vi "Create Data Class.vi"(8 "error in (no error)":errorcluster) -> (0 "error out":errorcluster, 3 "DVR":refnum<data-value>)   [LabVIEW 2022 SP3, in "XY Stage Data Class.lvclass"]
uses:
  XY Stage Data Class.lvclass
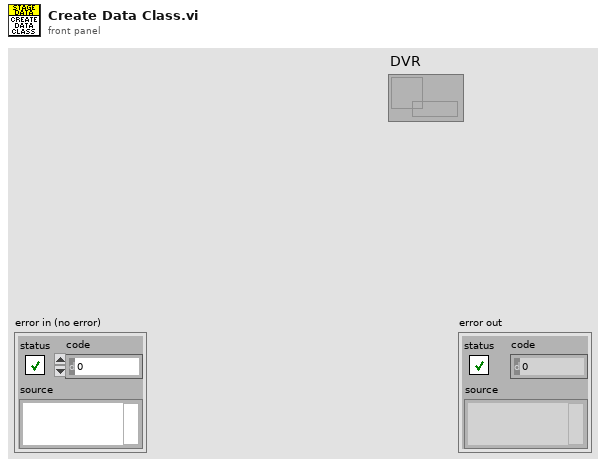
[diagram p1: front panel]
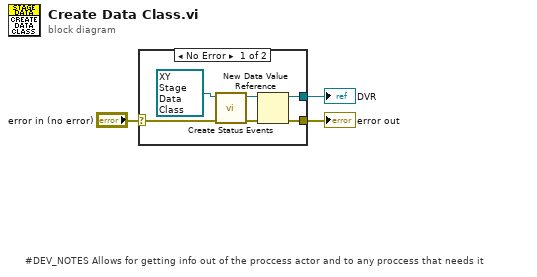
[diagram p0: block diagram]
diagram:
  # "#DEV_NOTES Allows for getting info out of the proccess actor and to any proccess that needs it"
  n1 = case shown="No Error" "error in (no error)" {
    selector: "error in (no error)" -> [w5 w10]
    tunnel: [w8 w10] -> w2
    tunnel: [w7 _] -> w1
    frame No Error {
      n2 = call "Create Status Events.vi"("error in (no error)"=w5, "XY Stage Data Class in"=refnum<class "XY Stage Data Class.lvclass"> refnum) -> ("error out"=w4:errorcluster, "XY Stage Data Class out"=w6:refnum<class "XY Stage Data Class.lvclass">)  [unwired: 8 in]
      n3 = New Data Value Reference(data value=w6, error in=w4) -> (data value reference=w7:refnum<data-value>, error out=w8:errorcluster)
    }
    frame Error {
    }
  }
  "error out" <- w2
  "DVR" <- w1
